vi "Ask XY.vi"(8 "error in (no error)":errorcluster, 11 "Module in":refnum<class "Module.lvclass">) -> (0 "error out":errorcluster, 1 "Y Error Out":dbl, 2 "X Error Out":dbl, 3 "Module out":refnum<class "Module.lvclass">)   [LabVIEW 2018, in "Module.lvclass"]
uses:
  Module.lvclass
  Module.lvclass/Module.ctl
panel:
  in  "Y Error":dbl
  in  "Submit":bool
  in  "X Error":dbl
  out "Tray Number":dbl
  out "Tray Region":dbl
  out "Tray Position":dbl
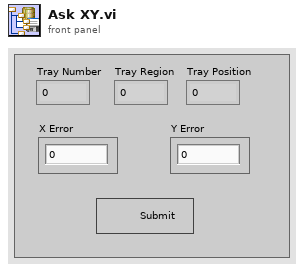
[diagram p1: front panel]
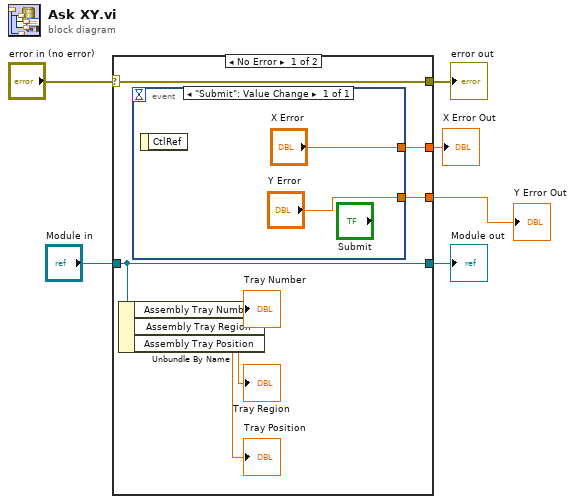
[diagram p0: block diagram]
diagram:
  n1 = case shown="No Error" "error in (no error)" {
    selector: "error in (no error)" -> [w13 w17]
    tunnel: [w13 w17] -> w3
    tunnel: [w12 w16] -> w5
    tunnel: "Module in" -> [w12 w16]
    tunnel: [w8 _] -> w1
    tunnel: [w7 _] -> w2
    frame No Error {
      n2 = Unbundle By Name(w12) -> ("Assembly Tray Number"=→"Tray Number":dbl, "Assembly Tray Region"=→"Tray Region":dbl, "Assembly Tray Position"=→"Tray Position":dbl)
      n3 = event shown="[0] \"Submit\": Value Change" {
        selector: _ -> [_]
        dyn-events: _ -> [_]
        timeout: _ -> [_]
        tunnel: ["X Error"] -> w8
        tunnel: ["Y Error"] -> w7
        event "Submit": Value Change {
          n4 = event-data() -> ()  [unwired: 1 in, 1 out]
        }
      }
    }
    frame Error {
    }
  }
  "error out" <- w3
  "Module out" <- w5
  "X Error Out" <- w1
  "Y Error Out" <- w2
